vi "rotate_about_prinicipal_axis.vi"(8 "error in (no error)":errorcluster, 9 "angle":dbl[unit], 10 "axis":T1, 11 "GenericTrajectory in":refnum<class "TrajectoryDL091126GenericVoxel.lvclass">) -> (0 "error out":errorcluster, 3 "GenericTrajectory out":refnum<class "TrajectoryDL091126GenericVoxel.lvclass">)   [LabVIEW 2010, in "TrajectoryDL091126GenericVoxel.lvclass"]
uses:
  TrajectoryDL091126GenericVoxel.lvclass
  common/legacy/axes.ctl
  common/enumerations/x_y_z_enumeration.ctl
  common/enumerations/functional_global_action_enum.ctl
  <vilib>/Analysis/Matrix/Numeric/Conversions/Array To Matrix - RA2.vi
  <vilib>/Analysis/baseanly.llb/Real A x B.vi
  common/classes/ErrorController/ErrorController/class_data.vi
  <vilib>/Analysis/Matrix/NI_Matrix.lvlib
  <vilib>/Analysis/NI_AALBase.lvlib
  common/classes/ErrorController/ErrorController/ErrorController.lvclass
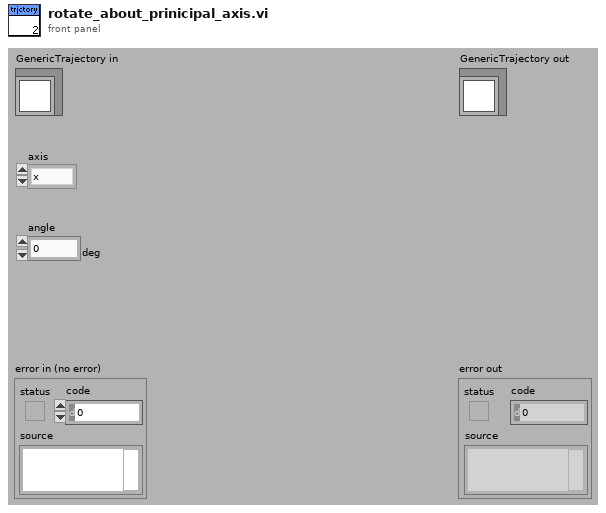
[diagram p1: front panel]
types:
  T1 = typedef "axes.ctl" = enum16{"x", "y", "z"}
  T2 = typedef "x_y_z_enumeration.ctl" = enum16{"x", "y", "z"}
  T3 = typedef "functional_global_action_enum.ctl" = enum16{"get", "set", "reset"}
  T4 = typedef "NI_Matrix.lvlib/RealMatrix.ctl" = dbl[][]
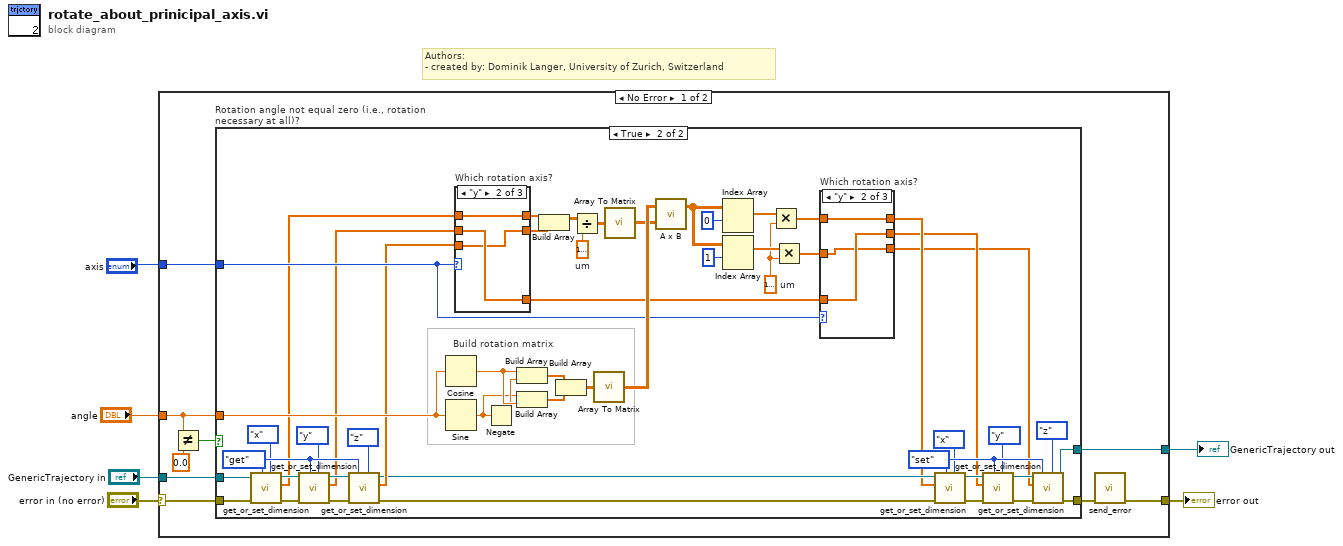
[diagram p0: block diagram]
diagram:
  # "Authors: \n- created by: Dominik Langer, University of Zurich, Switzerland"
  n1 = case shown="No Error" "error in (no error)" {
    selector: "error in (no error)" -> [w14 w89]
    tunnel: [w8 w89] -> w5
    tunnel: [w10 w88] -> w4
    tunnel: "angle" -> [w12 _]
    tunnel: "axis" -> [w11 _]
    tunnel: "GenericTrajectory in" -> [w9 w88]
    frame No Error {
      n2 = Not Equal?(x=w12, y=dbl[unit] 0.0) -> (x != y?=w13:bool)
      n3 = case "Rotation angle not equal zero (i.e., rotation necessary at all)?" shown="True" w13 {
        tunnel: w14 -> [w17 w45]
        tunnel: w12 -> [_ w47]
        tunnel: w11 -> [_ w46]
        tunnel: [w17 w29] -> w7
        tunnel: [w16 w27] -> w10
        tunnel: w9 -> [w16 w44]
        frame False {
        }
        frame True {
          w35 = functional_global_action_enum."set" ("action")
          w39 = functional_global_action_enum."get" ("action")
          w50 = dbl[unit] 1e-06  # um
          w55 = dbl[unit] 1e-06  # um
          # "Build rotation matrix"
          n4 = call-dynamic "get_or_set_dimension.vi"("dimension"=x_y_z_enumeration."x", "action"=w39, "error in (no error)"=w45, "GenericTrajectory in"=w44) -> ("error out"=w42:errorcluster, "pixel values out (single dimension)"=w36:dbl[unit][], "GenericTrajectory out"=w41:refnum<class "TrajectoryDL091126GenericVoxel.lvclass">)  [unwired: 2 in, 3 out]
          n5 = call-dynamic "get_or_set_dimension.vi"("dimension"=x_y_z_enumeration."y", "action"=w39, "error in (no error)"=w42, "GenericTrajectory in"=w41) -> ("error out"=w43:errorcluster, "pixel values out (single dimension)"=w37:dbl[unit][], "GenericTrajectory out"=w40:refnum<class "TrajectoryDL091126GenericVoxel.lvclass">)  [unwired: 2 in, 3 out]
          n6 = call-dynamic "get_or_set_dimension.vi"("dimension"=x_y_z_enumeration."z", "action"=w39, "error in (no error)"=w43, "GenericTrajectory in"=w40) -> ("error out"=w30:errorcluster, "pixel values out (single dimension)"=w38:dbl[unit][], "GenericTrajectory out"=w28:refnum<class "TrajectoryDL091126GenericVoxel.lvclass">)  [unwired: 2 in, 3 out]
          n7 = Cosine(x=w47) -> (cos(x)=w66:dbl)
          n8 = Sine(x=w47) -> (sin(x)=w64:dbl)
          n9 = case "Which rotation axis?" shown="\"y\"" w46 {
            tunnel: [w80 w83 w87] -> w59
            tunnel: w36 -> [w81 w83 w87]
            tunnel: [w79 w82 w86] -> w58
            tunnel: w37 -> [w80 w84 w86]
            tunnel: [w81 w84 w85] -> w53
            tunnel: w38 -> [w79 w82 w85]
            frame "x", Default {
            }
            frame "y" {
            }
            frame "z" {
            }
          }
          n10 = Negate(x=w64) -> (-x=w65:dbl)
          n11 = Build Array(w66, w65) -> (w69:dbl[])
          n12 = Build Array(w64, w66) -> (w68:dbl[])
          n13 = Build Array(w59, w58) -> (w56:dbl[unit][][])
          n14 = Build Array(w69, w68) -> (w67:dbl[][])
          n15 = Divide(x=w56, y=w55) -> (x/y=w54:dbl[][])
          n16 = call-poly <vilib>:"Array To Matrix.vi"("Real 2D Array"=w67) -> ("Real Matrix"=w60:T4)
          n17 = call-poly <vilib>:"Array To Matrix.vi"("Real 2D Array"=w54) -> ("Real Matrix"=w57:T4)
          n18 = call-poly <vilib>:"A x B.vi"("B"=w57, "A"=w60) -> ("A x B"=w61:T4)  [unwired: 1 out]
          n19 = Index Array(array=w61, index (row)=0) -> (element=w52:dbl[])  [unwired: 1 in]
          n20 = Index Array(array=w61, index (row)=1) -> (element=w51:dbl[])  [unwired: 1 in]
          n21 = Multiply(x=w52, y=w50) -> (x*y=w49:dbl[unit][])
          n22 = Multiply(x=w51, y=w50) -> (x*y=w48:dbl[unit][])
          n23 = case "Which rotation axis?" shown="\"y\"" w46 {
            tunnel: [w72 w74 w78] -> w26
            tunnel: w49 -> [w71 w74 w78]
            tunnel: [w71 w75 w77] -> w25
            tunnel: w48 -> [w70 w73 w77]
            tunnel: [w70 w73 w76] -> w24
            tunnel: w53 -> [w72 w75 w76]
            frame "x", Default {
            }
            frame "y" {
            }
            frame "z" {
            }
          }
          n24 = call-dynamic "get_or_set_dimension.vi"("dimension"=x_y_z_enumeration."x", "action"=w35, "error in (no error)"=w30, "pixel values in (single dimension)"=w26, "GenericTrajectory in"=w28) -> ("error out"=w32:errorcluster, "GenericTrajectory out"=w33:refnum<class "TrajectoryDL091126GenericVoxel.lvclass">)  [unwired: 1 in, 4 out]
          n25 = call-dynamic "get_or_set_dimension.vi"("dimension"=x_y_z_enumeration."y", "action"=w35, "error in (no error)"=w32, "pixel values in (single dimension)"=w25, "GenericTrajectory in"=w33) -> ("error out"=w31:errorcluster, "GenericTrajectory out"=w34:refnum<class "TrajectoryDL091126GenericVoxel.lvclass">)  [unwired: 1 in, 4 out]
          n26 = call-dynamic "get_or_set_dimension.vi"("dimension"=x_y_z_enumeration."z", "action"=w35, "error in (no error)"=w31, "pixel values in (single dimension)"=w24, "GenericTrajectory in"=w34) -> ("error out"=w29:errorcluster, "GenericTrajectory out"=w27:refnum<class "TrajectoryDL091126GenericVoxel.lvclass">)  [unwired: 1 in, 4 out]
        }
      }
      n27 = call "send_error.vi"("error in (no error)"=w7) -> ("error out"=w8:errorcluster)  [unwired: 10 in]
    }
    frame Error {
    }
  }
  "error out" <- w5
  "GenericTrajectory out" <- w4
